vi "Connection Open Tree.vi"(8 "error in (no error)":errorcluster, 9 "Shot":i32, 10 "Tree":string, 11 "Connection DVR in":refnum<data-value>) -> (0 "error out":errorcluster, 3 "Connection DVR out":refnum<data-value>)   [LabVIEW 2015, in "MDSplus.lvlib"]
uses:
  <vilib>/MDSplus/Library/MDSplus.lvlib
  <vilib>/MDSplus/Classes/Connection_Class/Connection.lvclass
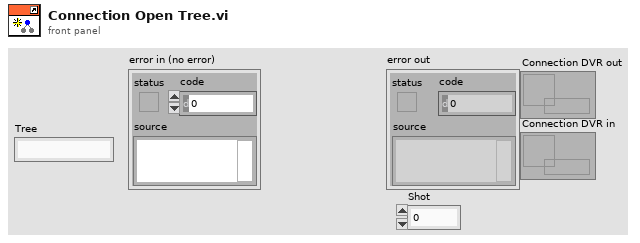
[diagram p1: front panel]
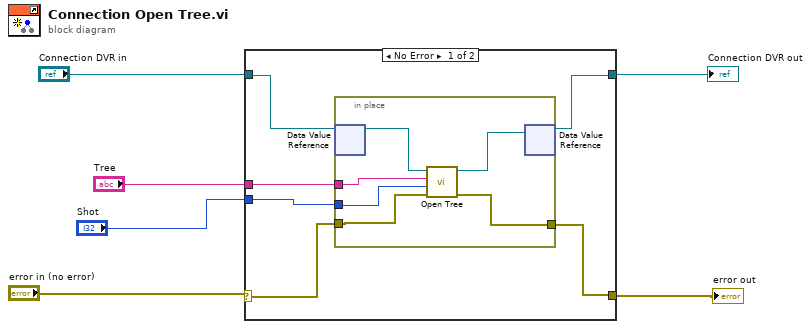
[diagram p0: block diagram]
diagram:
  n1 = case shown="No Error" "error in (no error)" {
    selector: "error in (no error)" -> [w9 w19]
    tunnel: "Connection DVR in" -> [w12 w20]
    tunnel: [w11 w20] -> w4
    tunnel: [w7 w19] -> w3
    tunnel: "Tree" -> [w10 _]
    tunnel: "Shot" -> [w8 _]
    frame No Error {
      n2 = in-place {
        in-place-border: w10 -> [w14]
        in-place-border: w9 -> [w16]
        in-place-border: w8 -> [w13]
        in-place-border: [w15] -> w7
        n3 = in-place-dvr #1(w12) -> (w18:refnum<class "Connection.lvclass">)  [unwired: 1 out]
        n4 = call <vilib>:"Open Tree.vi"("error in (no error)"=w16, "Shot"=w13, "Tree"=w14, "Connection in"=w18) -> ("error out"=w15:errorcluster, "Connection out"=w17:refnum<class "Connection.lvclass">)  [unwired: 6 in]
        n5 = in-place-dvr #1(w17) -> (w11:refnum<data-value>)  [unwired: 1 out]
      }
    }
    frame Error {
    }
  }
  "error out" <- w3
  "Connection DVR out" <- w4
